vi "Spindle_speed_RT (SubVI).vi"(11 "String":string) -> (0 "error out":errorcluster, 1 "content 4":string, 2 "content1 2":string, 3 "after match 2":string, 4 "empty? 2":bool, 5 "concatenated string":string, 6 "spindle speed":string, 7 "concatenated string 2":string)   [LabVIEW 2017]
uses:
  MT_connect_data.ctl
  <vilib>/regexp/Match Regular Expression.xnode
  <vilib>/addons/internet/NI_InternetTK_Core_VIs.lvlib
panel:
  in  "?":T1
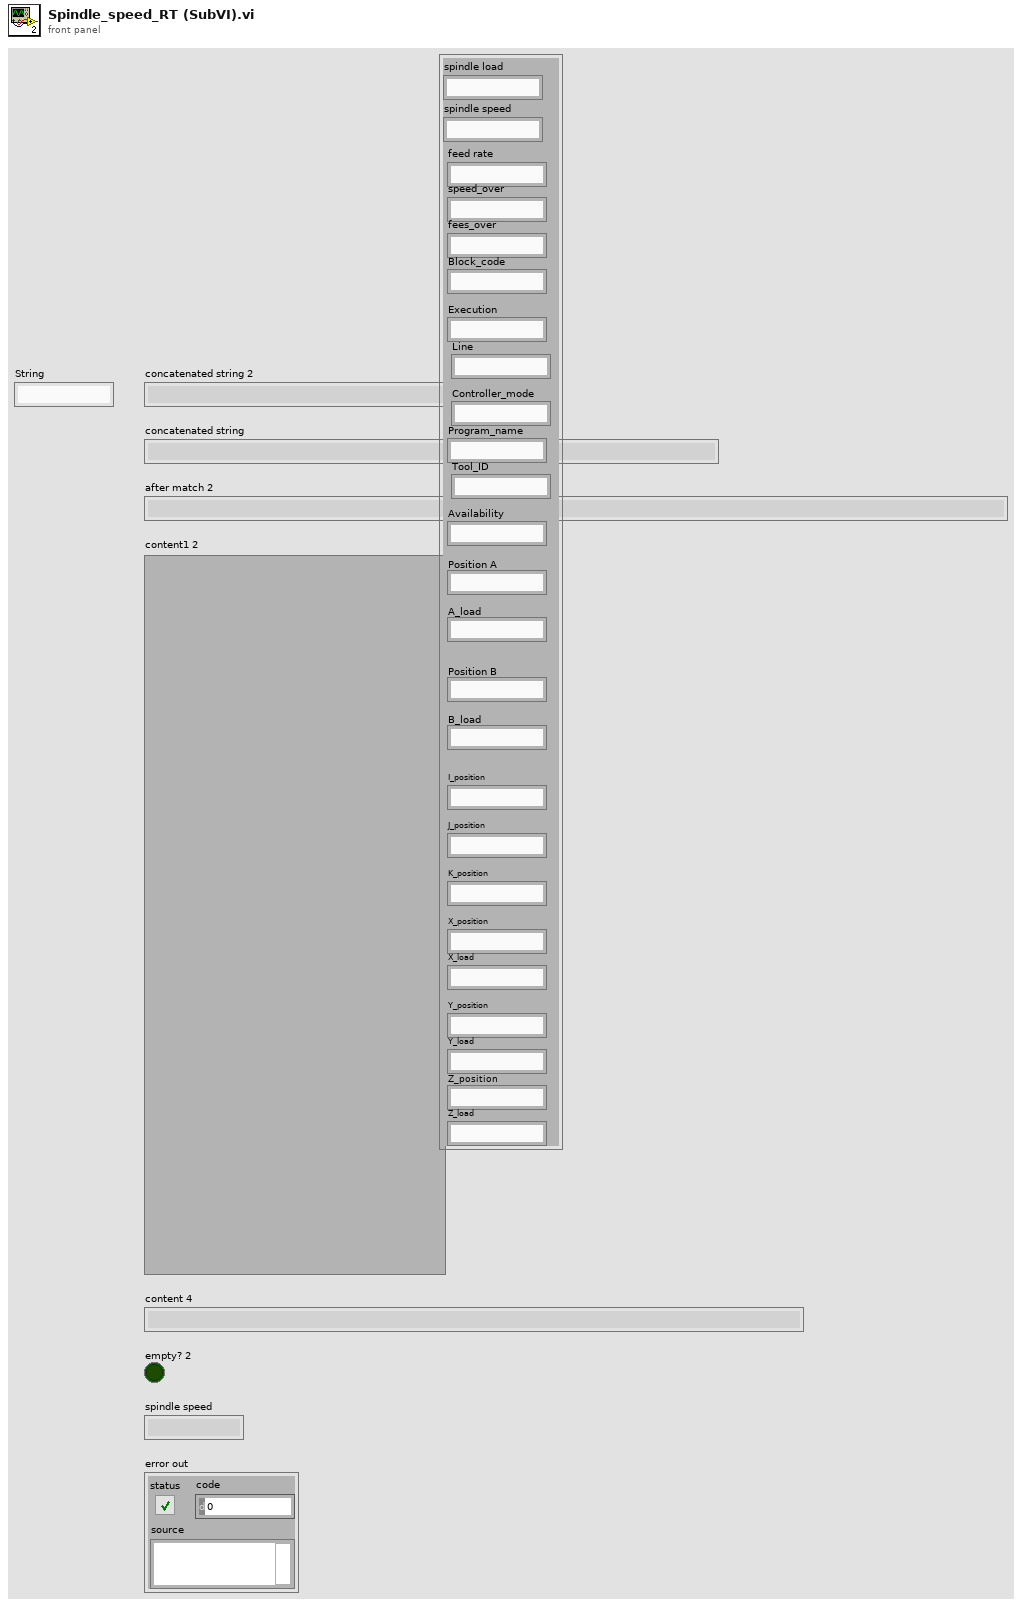
[diagram p1: front panel]
types:
  T1 = typedef "MT_connect_data.ctl" = cluster{"spindle load ":string, "spindle speed ":string, "feed rate":string, "speed_over":string, "fees_over":string, "Block_code":string, "Execution":string, "Line":string, "Controller_mode":string, "Program_name":string, "Tool_ID":string, "Availability":string, "Position A":string, "A_load":string, "Position B":string, "B_load":string, "I_position":string, "J_position":string, "K_position":string, "X_position":string, "X_load":string, "Y_position":string, "Y_load":string, "Z_position":string, "Z_load":string}
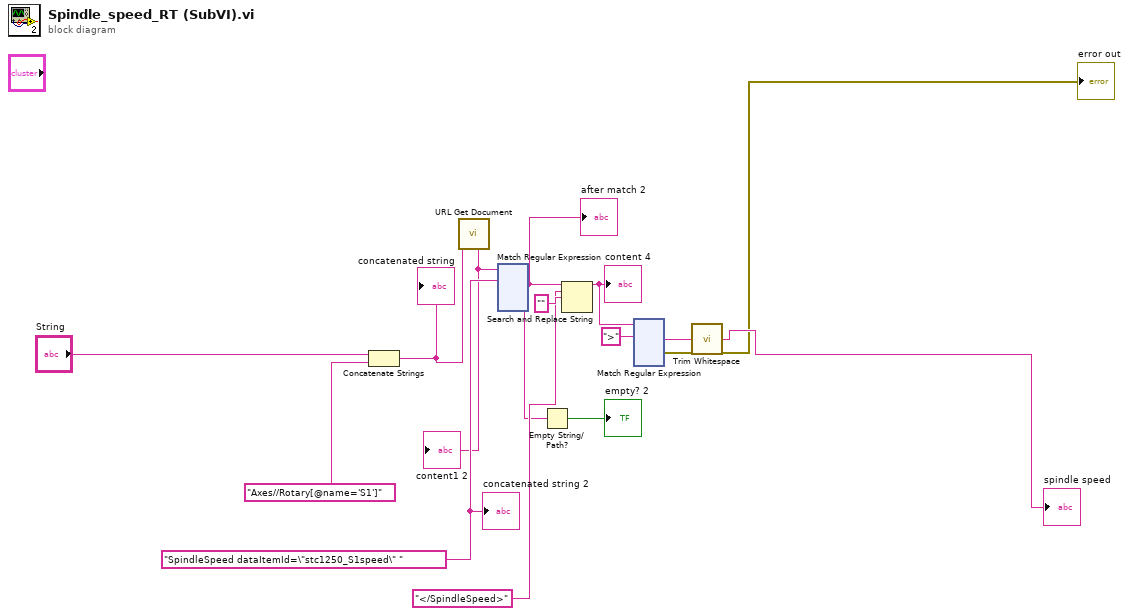
[diagram p0: block diagram]
diagram:
  w12 = "SpindleSpeed dataItemId=\"stc1250_S1speed\" " ("regular expression")
  n1 = Concatenate Strings("String", "Axes//Rotary[@name='S1']" ("string")) -> (w7:string)
  "concatenated string" <- w7
  n2 = call <vilib>:"URL Get Document.vi"("URL"=w7) -> ("content"=w4:string)  [unwired: 6 in, 4 out]
  "content1 2" <- w4
  n3 = xnode "Match Regular Expression"("input string"=w4, "regular expression"=w12) -> ("after match"=w3:string, "submatch 1"=w6:string)  [unwired: 4 in, 4 out]
  "after match 2" <- w3
  n4 = Empty String/Path?(string/path=w6) -> (empty?=→"empty? 2":bool)
  n5 = Search and Replace String(input string=w3, search string="</SpindleSpeed>" ("string"), replace string="" ("string")) -> (result string=w2:string)  [unwired: 5 in, 3 out]
  "content 4" <- w2
  n6 = xnode "Match Regular Expression"("input string"=w2, "regular expression"=">" ("string")) -> ("after match"=w1:string, "error out"=→"error out":errorcluster)  [unwired: 4 in, 4 out]
  n7 = call <vilib>:"Trim Whitespace.vi"("string"=w1) -> ("trimmed string"=→"spindle speed":string)  [unwired: 1 in]
  "concatenated string 2" <- w12
